vi "PCO_Init.vi"(8 "entrée d'erreur (pas d'erreur)":errorcluster) -> (0 "sortie d'erreur":errorcluster, 3 "Camera en sortie":refnum<class "Camera.lvclass">)   [LabVIEW 2026]
uses:
  pco.labview/camera/Camera.lvclass
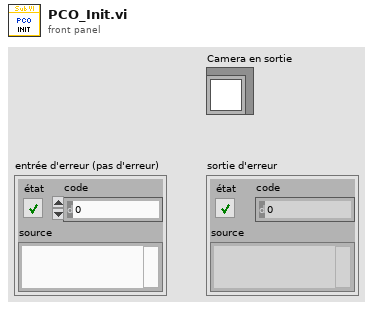
[diagram p1: front panel]
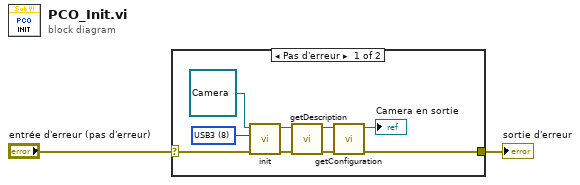
[diagram p0: block diagram]
diagram:
  n1 = case shown="Pas d'erreur" "entrée d'erreur (pas d'erreur)" {
    selector: "entrée d'erreur (pas d'erreur)" -> [w5 w12]
    tunnel: [w11 w12] -> w2
    frame No Error {
      w7 = u16 8 items=["FireWire"=1, "GenICam"=3, "GigE"=5, "USB"=6, "CameraLinkME4"=7, "USB3"=8, "CLHS"=11, "All"=65535] ("interface")
      n2 = call-dynamic "init.vi"("Camera in"=refnum<class "Camera.lvclass"> refnum, "interface"=w7, "error in (no error)"=w5) -> ("Camera out"=w4:refnum<class "Camera.lvclass">, "error out"=w3:errorcluster)  [unwired: 6 in]
      n3 = call-dynamic "getDescription.vi"("error in (no error)"=w3, "Camera in"=w4) -> ("error out"=w10:errorcluster, "Camera out"=w8:refnum<class "Camera.lvclass">)  [unwired: 7 in, 1 out]
      n4 = call-dynamic "getConfiguration.vi"("error in (no error)"=w10, "Camera in"=w8) -> ("error out"=w11:errorcluster, "Camera out"=→"Camera en sortie":refnum<class "Camera.lvclass">)  [unwired: 7 in, 1 out]
    }
    frame Error {
    }
  }
  "sortie d'erreur" <- w2
